vi "Seq Change Data type.vi"(8 "Error in":errorcluster, 10 "DO Seq in":T1(array[cluster]), 11 "AO Seq in":T1(array[cluster])) -> (0 "Error out":errorcluster, 2 "AO":T2(array[cluster]), 3 "DO":T3(array[cluster]))   [LabVIEW 2022 SP3]
uses:
  59f8556c-de76-4912-9bab-8612dc492592.vi
  c5ed2412-1fc7-491a-b1ad-bc940cd6d3e0.vi
  <vilib>/Comparison/Less/Less Functor/Less Functor.lvclass
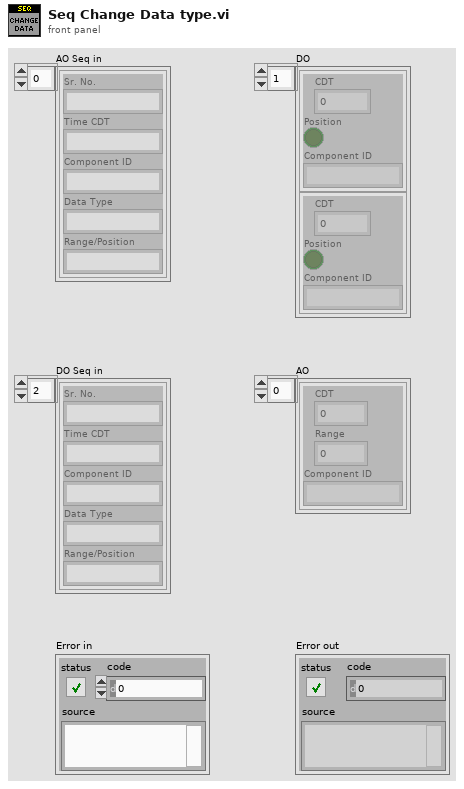
[diagram p1: front panel]
types:
  T1 = cluster{"Sr. No.":string, "Time CDT":string, "Component ID":string, "Data Type":string, "Range/Position":string}[]
  T2 = cluster{"CDT":dbl, "Range":dbl, "Component ID":string}[]
  T3 = cluster{"CDT":dbl, "Position":bool, "Component ID":string}[]
  T4 = cluster{"CDT":dbl, "Position":bool, "Component ID":string}
  T5 = cluster{"CDT":dbl, "Range":dbl, "Component ID":string}
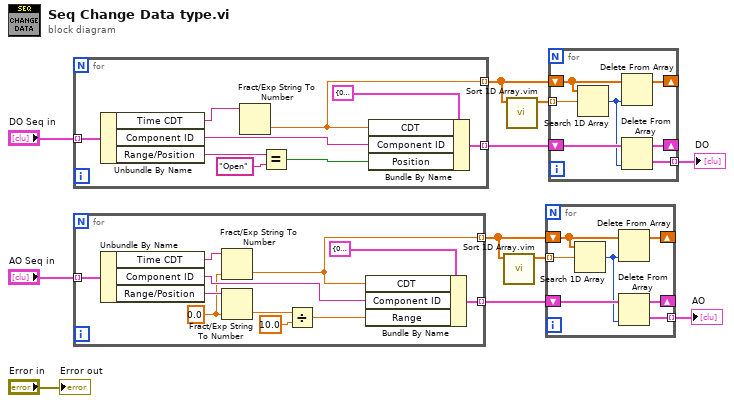
[diagram p0: block diagram]
diagram:
  n1 = for {
    tunnel: "DO Seq in" -> [w20] mode=indexing
    tunnel: [w13] -> w8 mode=indexing
    tunnel: [w12] -> w7 mode=indexing
    n2 = Unbundle By Name(w20) -> ("Time CDT"=w19:string, "Component ID"=w17:string, "Range/Position"=w16:string)
    n3 = Fract/Exp String To Number(string=w19) -> (number=w12:dbl)  [unwired: 3 in, 1 out]
    n4 = Equal?(x=w16, y="Open") -> (x = y?=w14:bool)
    n5 = Bundle By Name(cluster=T4 {"CDT"=0.0, "Position"=TRUE, "Component ID"=""}, "CDT"=w12, "Component ID"=w17, "Position"=w14) -> (w13:T4)
  }
  n6 = for {
    tunnel: "AO Seq in" -> [w31] mode=indexing
    tunnel: [w27] -> w2 mode=indexing
    tunnel: [w24] -> w3 mode=indexing
    w25 = 0.0 ("default (0 I32)")
    n7 = Unbundle By Name(w31) -> ("Time CDT"=w30:string, "Component ID"=w28:string, "Range/Position"=w26:string)
    n8 = Fract/Exp String To Number(string=w30, default (0 dbl)=w25) -> (number=w24:dbl)  [unwired: 2 in, 1 out]
    n9 = Fract/Exp String To Number(string=w26, default (0 dbl)=w25) -> (number=w23:dbl)  [unwired: 2 in, 1 out]
    n10 = Divide(x=w23, y=10.0) -> (x/y=w21:dbl)
    n11 = Bundle By Name(cluster=T5 {"CDT"=0.0, "Range"=0.0, "Component ID"=""}, "CDT"=w24, "Component ID"=w28, "Range"=w21) -> (w27:T5)
  }
  n12 = call "Sort 1D Array.vim"("unsorted array"=w3) -> ("sorted array"=w1:dbl[])  [unwired: 10 in]
  n13 = call "Sort 1D Array.vim"("unsorted array"=w7) -> ("sorted array"=w6:dbl[])  [unwired: 10 in]
  n14 = for {
    tunnel: w1 -> [w37] mode=indexing
    tunnel: [w36] -> w4 mode=indexing
    shift-right: [w33] -> _
    shift-left: w3 -> [w35]
    shift-right: [w32] -> _
    shift-left: w2 -> [w38]
    n15 = Search 1D Array(1D array=w35, element=w37) -> (index of element=w34:i32)  [unwired: 1 in]
    n16 = Delete From Array(array=w35, index=w34) -> (array with subset deleted=w33:dbl[])  [unwired: 1 in, 1 out]
    n17 = Delete From Array(array=w38, index=w34) -> (deleted portion=w36:T5, array with subset deleted=w32:T2)  [unwired: 1 in]
  }
  "AO" <- w4
  n18 = for {
    tunnel: w6 -> [w44] mode=indexing
    tunnel: [w43] -> w5 mode=indexing
    shift-right: [w40] -> _
    shift-left: w7 -> [w42]
    shift-right: [w39] -> _
    shift-left: w8 -> [w45]
    n19 = Search 1D Array(1D array=w42, element=w44) -> (index of element=w41:i32)  [unwired: 1 in]
    n20 = Delete From Array(array=w42, index=w41) -> (array with subset deleted=w40:dbl[])  [unwired: 1 in, 1 out]
    n21 = Delete From Array(array=w45, index=w41) -> (deleted portion=w43:T4, array with subset deleted=w39:T3)  [unwired: 1 in]
  }
  "DO" <- w5
  "Error out" <- "Error in"
